vi "Resolve URL.vi"(8 "error in (no error)":errorcluster, 10 "Path":string, 11 "REST Client in":refnum<class "REST Client.lvclass">) -> (0 "error out":errorcluster, 2 "Resolved URL":string, 3 "REST Client out":refnum<class "REST Client.lvclass">)   [LabVIEW 2013, in "REST Client.lvlib" / "REST Client.lvclass"]
uses:
  REST Client.lvclass
  REST Client.lvclass/REST Client.ctl
  <vilib>/wsapi/NI_WebServices.lvlib
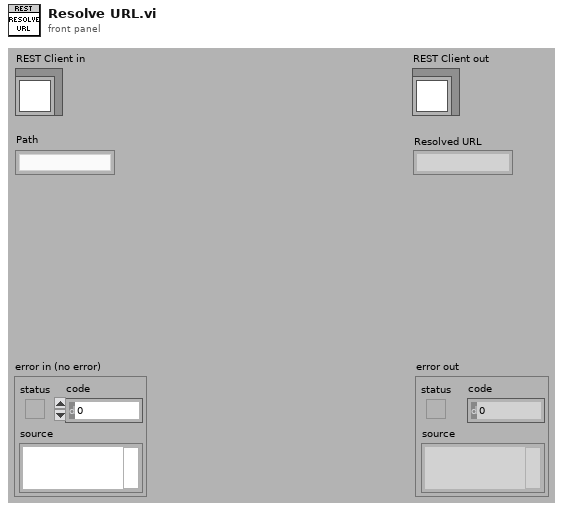
[diagram p1: front panel]
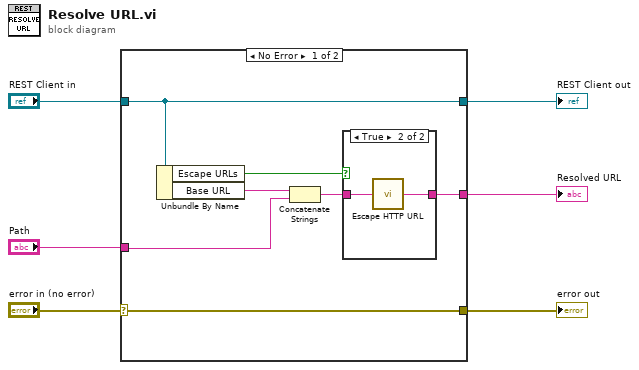
[diagram p0: block diagram]
diagram:
  n1 = case shown="No Error" "error in (no error)" {
    selector: "error in (no error)" -> [w8 w18]
    tunnel: [w8 w18] -> w5
    tunnel: [w9 w17] -> w3
    tunnel: "REST Client in" -> [w9 w17]
    tunnel: "Path" -> [w13 _]
    tunnel: [w11 _] -> w1
    frame No Error {
      n2 = Unbundle By Name(w9) -> ("Escape URLs"=w7:bool, "Base URL"=w10:string)
      n3 = Concatenate Strings(w10, w13) -> (w12:string)
      n4 = case shown="True" w7 {
        tunnel: w12 -> [w14 w16]
        tunnel: [w14 w15] -> w11
        frame False {
        }
        frame True {
          n5 = call <vilib>:"Escape HTTP URL.vi"("unescaped string in"=w16) -> ("escaped string out"=w15:string)
        }
      }
    }
    frame Error {
    }
  }
  "error out" <- w5
  "REST Client out" <- w3
  "Resolved URL" <- w1
